vi "GetPersistentConfiguration.vi"(8 "Error In":errorcluster, 9 "DataIn":variant, 11 "object in":refnum<class "ITAFObject.lvclass">) -> (0 "Error Out":errorcluster, 1 "DataOut":variant, 3 "object out":refnum<class "ITAFObject.lvclass">)   [LabVIEW 2021, in "ITAFObject.lvclass"]
uses:
  ITAFObject.lvclass
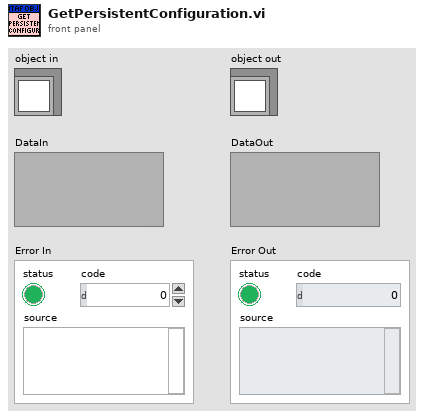
[diagram p1: front panel]
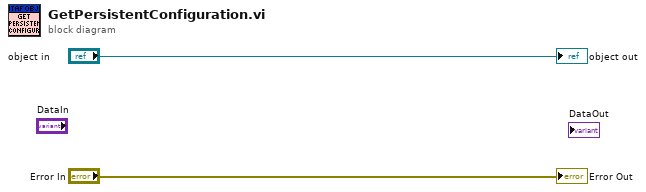
[diagram p0: block diagram]
diagram:
  "Error Out" <- "Error In"
  "object out" <- "object in"
